vi "Reset EtherCAT Chassis after connection Loss.vi"   [LabVIEW 2012]
doc: "This VI dsemonstrates how to reset the EtherCAT chassis after experiencing a connection loss."
panel:
  # "Overview: Demonstrates how to  reset the EtherCAT chassis after experiencing a connection loss. \n\nRequirements: LabVIEW Base Development System 2012 (or compatible)\n                          LabVIEW Real-Time Module 2012 (or compatible)\n                          NI-RIO 12.0 (or compatible)\n                          NI-Industrial Communications for EtherCAT 2.4 (or compatible)\n\nInstructions: \n1. Run the VI\n2. (Optional) Disconnect the ethernet cable from the 9144 chassis."
types:
  T1 = enum16{"shutdown", "Working code", "Error Handle"}
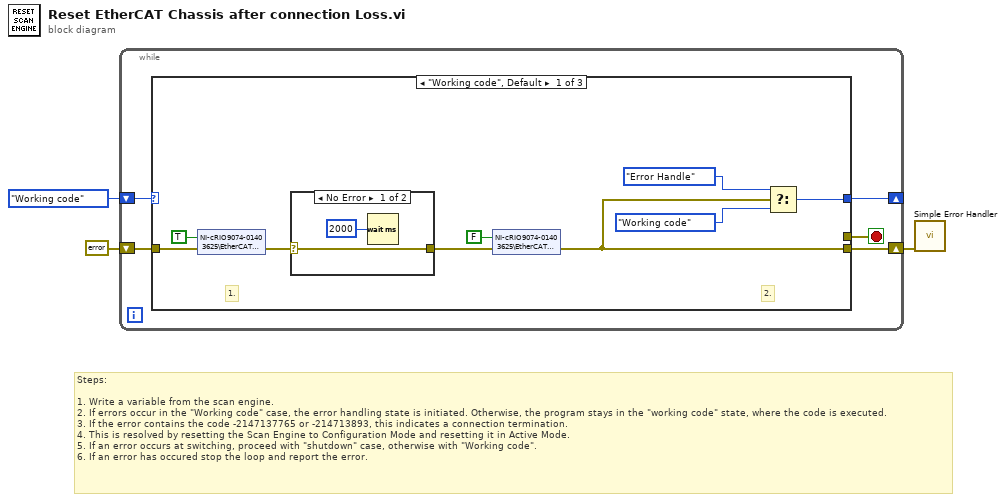
[diagram p0: block diagram]
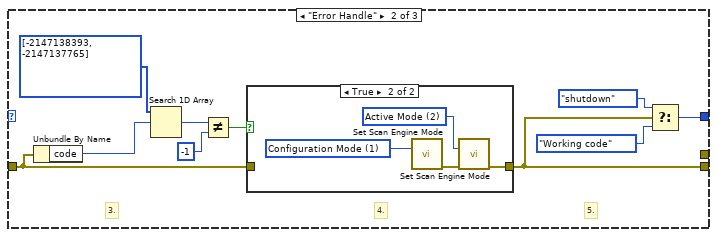
[diagram p3: hidden frame]
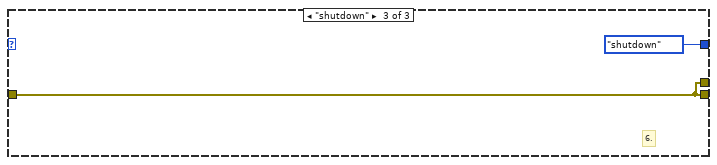
[diagram p5: hidden frame]
diagram:
  # "Steps:\n\n1. Write a variable from the scan engine.\n2. If errors occur in the \"Working code\" case, the error handling state is initiated. Otherwise, the program stays in the \"working code\" state, where the code is executed.\n3. If the error contains the code -2147137765 or -214713893, this indicates a connection termination.\n4. This is resolved by resetting the Scan Engine to Configuration Mode and resetting it in Active Mode.\n5. If an error occurs at switching, proceed with \"shutdown\" case, otherwise with \"Working code\".\n6. If an error has occured stop the loop and report the error."
  n1 = while {
    shift-right: [w8] -> w2
    shift-left: errorcluster {"status"=FALSE, "code"=0, "source"=""} ("error out") -> [w6]
    shift-right: [w5] -> _
    shift-left: T1."Working code" -> [w7]
    stop <- w4 stop-if-true
    n2 = case shown="\"Working code\", Default" w7 {
      tunnel: [w9 w23 w37] -> w8
      tunnel: w6 -> [w13 w21 w37]
      tunnel: [w10 w24 T1."shutdown"] -> w5
      tunnel: [_ _ w37] -> w4
      frame "Working code", Default {
        # "2."
        # "1."
        n3 = shared-variable "NI-cRIO9074-01403625\\EtherCAT Master\\Device\\Mod1\\DO0"(TRUE ("DO0"), error in=w13) -> (error out=w15:errorcluster)
        n4 = case shown="No Error" w15 {
          selector: w15 -> [w19 w20]
          tunnel: [w19 w20] -> w14
          frame No Error {
            n5 = Wait (ms)(milliseconds to wait=u32 2000) -> ()  [unwired: 1 out]
          }
          frame Error {
          }
        }
        n6 = shared-variable "NI-cRIO9074-01403625\\EtherCAT Master\\Device\\Mod1\\DO0"(FALSE ("DO0"), error in=w14) -> (error out=w9:errorcluster)
        n7 = Select(t=T1."Error Handle", s=w9, f=T1."Working code") -> (s? t:f=w10:T1)
      }
      frame "Error Handle" {
        # "5."
        # "4."
        # "3."
        n8 = Unbundle By Name(w21) -> ("code"=w29:i32)
        n9 = Search 1D Array(1D array=i32[] [-2147138393, -2147137765], element=w29) -> (index of element=w28:i32)  [unwired: 1 in]
        n10 = Not Equal?(x=w28, y=-1) -> (x != y?=w26:bool)
        n11 = case shown="True" w26 {
          tunnel: [w31 w32] -> w23
          tunnel: w21 -> [w31 _]
          frame False {
          }
          frame True {
            w33 = 2 items=["Configuration Mode"=1, "Active Mode"=2] ("mode (Active Mode)")
            w34 = 1 items=["Configuration Mode"=1, "Active Mode"=2] ("mode (Active Mode)")
            n12 = call <vilib>:"Set Scan Engine Mode.vi"("mode (Active Mode)"=w34) -> ("error out"=w35:errorcluster)  [unwired: 14 in]
            n13 = call <vilib>:"Set Scan Engine Mode.vi"("mode (Active Mode)"=w33, "error in (no error)"=w35) -> ("error out"=w32:errorcluster)  [unwired: 13 in]
          }
        }
        n14 = Select(t=T1."shutdown", s=w23, f=T1."Working code") -> (s? t:f=w24:T1)
      }
      frame "shutdown" {
        # "6."
      }
    }
  }
  n15 = call <vilib>:"Simple Error Handler.vi"("error in (no error)"=w2) -> ()  [unwired: 4 in, 5 out]
